vi "Apply Style.vi"(4 "header ref":refnum<vi>, 8 "error in":errorcluster, 9 "message ref":refnum<vi>, 10 "pop up ref":refnum<vi>, 11 "Theme in":refnum<class "Theme.lvclass">) -> (0 "error out":errorcluster, 3 "Theme out":refnum<class "Theme.lvclass">)   [LabVIEW 2021, in "Theme.lvclass"]
doc: "Apply the style to the message pop up : format the header, background, and message box\n\n<b>Code Developed By:</b> +\nDaniel Coons +\nhttps://github.com/danielcoons/tsc-pop-up"
uses:
  Theme.lvclass
  <vilib>/Utility/miscctls.llb/LVSelectionTypeDef.ctl
  Theme.lvclass/Theme.ctl
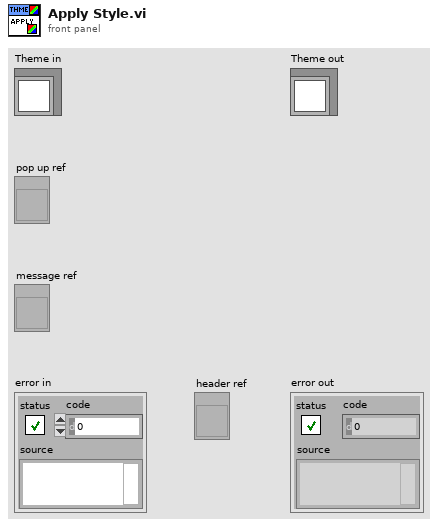
[diagram p1: front panel]
types:
  T1 = typedef "LVSelectionTypeDef.ctl" = cluster{"Selection Start":u32, "Selection End":u32}
  T2 = typedef "Theme.lvclass/message box--typdef.ctl" = cluster{"Text.Font Name":string, "Text.Font Size":u32, "Color":u32, "Text.Justification":enum16{"Left", "Center", "Right"}, "messge color":cluster{"border":u32, "fill":u32}}
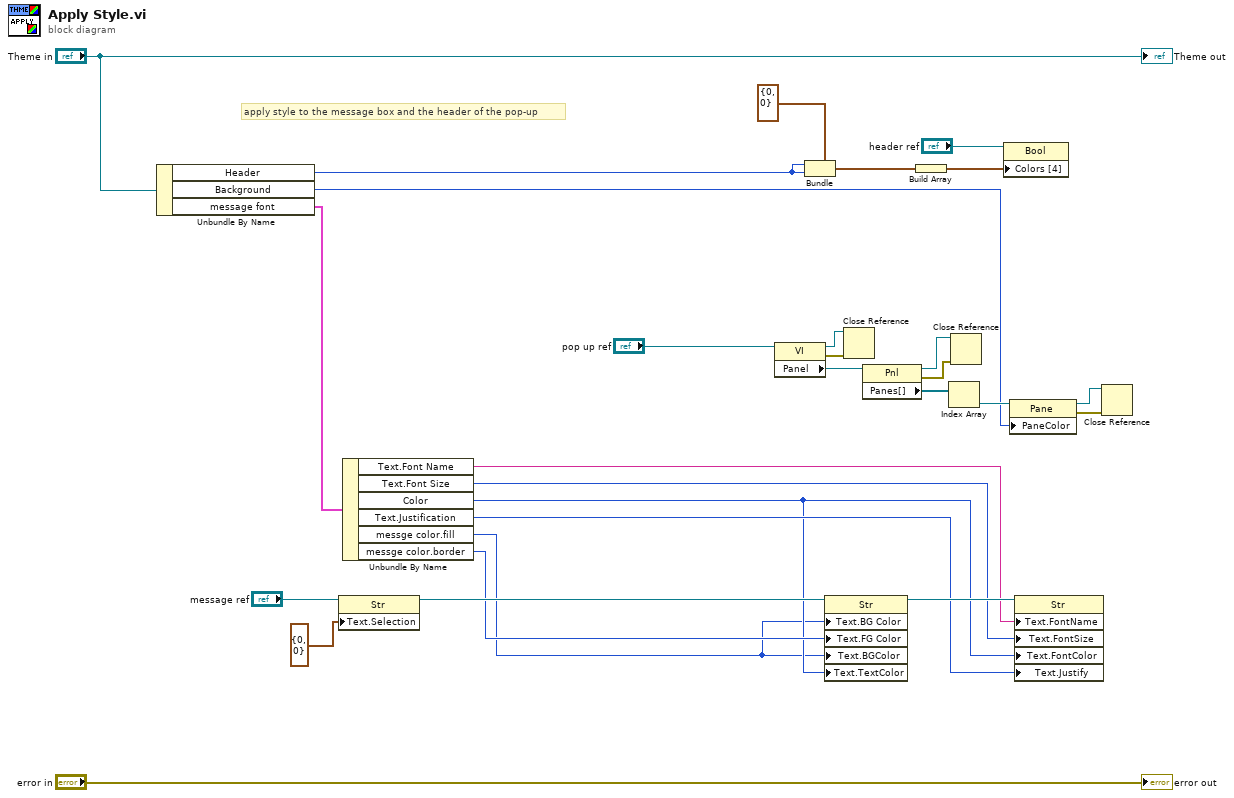
[diagram p0: block diagram]
diagram:
  # "apply style to the message box and the header of the pop-up"
  n1 = Unbundle By Name("Theme in") -> ("Header"=w18:u32, "Background"=w15:u32, "message font"=w12:T2)
  n2 = property on="Property Node" class="Str"(reference="message ref", "Text.Selection"=T1 {"Selection Start"=0, "Selection End"=0}) -> (reference out=w5:refnum<vi>)  [unwired: 1 in, 1 out]
  n3 = Unbundle By Name(w12) -> ("Text.Font Name"=w11:string, "Text.Font Size"=w10:u32, "Color"=w2:u32, "Text.Justification"=w9:enum16{"Left", "Center", "Right"}, "messge color.fill"=w1:u32, "messge color.border"=w3:u32)
  n4 = property on="Property Node" class="VI"(reference="pop up ref") -> (reference out=w6:refnum<vi>, error out=w26:errorcluster, "Panel"=w25:refnum<vi>)  [unwired: 1 in]
  n5 = Bundle(cluster=cluster{u32, u32} {0, 0}, w18, w18) -> (w17:cluster{u32, u32})
  n6 = property on="Property Node" class="Str"(reference=w5, "Text.BG Color"=w1, "Text.FG Color"=w3, "Text.BGColor"=w1, "Text.TextColor"=w2) -> (reference out=w13:refnum<vi>)  [unwired: 1 in, 1 out]
  n7 = Close Reference(reference=w6, error in (no error)=w26) -> ()  [unwired: 1 out]
  n8 = property on="Property Node" class="Pnl"(reference=w25) -> (reference out=w7:refnum<vi>, error out=w27:errorcluster, "Panes[]"=w24:refnum<vi>[])  [unwired: 1 in]
  n9 = Build Array(w17) -> (w16:cluster{u32, u32}[])
  n10 = Index Array(array=w24) -> (element=w23:refnum<vi>)  [unwired: 1 in]
  n11 = Close Reference(reference=w7, error in (no error)=w27) -> ()  [unwired: 1 out]
  n12 = property on="Property Node" class="Bool"(reference="header ref", "Colors [4]"=w16) -> ()  [unwired: 1 in, 2 out]
  n13 = property on="Property Node" class="Pane"(reference=w23, "PaneColor"=w15) -> (reference out=w8:refnum<vi>, error out=w28:errorcluster)  [unwired: 1 in]
  n14 = property on="Property Node" class="Str"(reference=w13, "Text.FontName"=w11, "Text.FontSize"=w10, "Text.FontColor"=w2, "Text.Justify"=w9) -> ()  [unwired: 1 in, 2 out]
  n15 = Close Reference(reference=w8, error in (no error)=w28) -> ()  [unwired: 1 out]
  "error out" <- "error in"
  "Theme out" <- "Theme in"
